vi "AlphaBetaToDQ_noSine.vi"(0 "alpha":sgl format="%#_32g", 1 "cosx":sgl, 2 "sinx":sgl, 5 "beta":sgl format="%#_32g", 12 "Resources":T1) -> (4 "direct":sgl, 6 "quadrature":sgl)   [LabVIEW 2017]
uses:
  Multiplier/Multiplier.lvclass
  Adder/Adder.lvclass
  Subtractor/Subtractor.lvclass
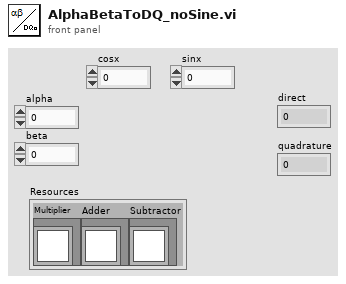
[diagram p1: front panel]
types:
  T1 = cluster{"Multiplier":refnum<class "Multiplier.lvclass">, "Adder":refnum<class "Adder.lvclass">, "Subtractor":refnum<class "Subtractor.lvclass">}
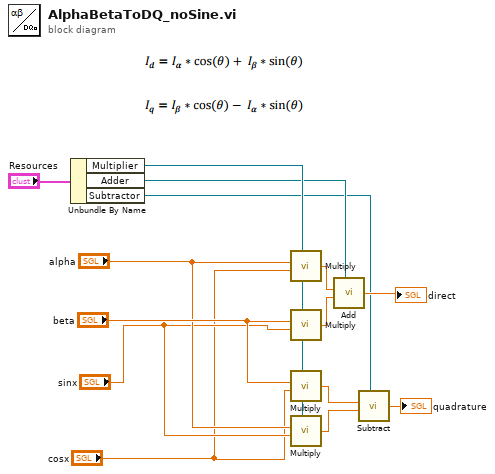
[diagram p0: block diagram]
diagram:
  n1 = Unbundle By Name("Resources") -> ("Multiplier"=w9:refnum<class "Multiplier.lvclass">, "Adder"=w2:refnum<class "Adder.lvclass">, "Subtractor"=w1:refnum<class "Subtractor.lvclass">)
  n2 = call-dynamic "Multiply.vi"("x"="alpha", "y"="cosx", "Multiplier"=w9) -> ("x*y"=w7:sgl)  [unwired: 4 in]
  n3 = call-dynamic "Multiply.vi"("x"="beta", "y"="sinx", "Multiplier"=w9) -> ("x*y"=w6:sgl)  [unwired: 4 in]
  n4 = call-dynamic "Multiply.vi"("x"="beta", "y"="cosx", "Multiplier"=w9) -> ("x*y"=w5:sgl)  [unwired: 4 in]
  n5 = call-dynamic "Multiply.vi"("x"="alpha", "y"="sinx", "Multiplier"=w9) -> ("x*y"=w4:sgl)  [unwired: 4 in]
  n6 = call-dynamic "Add.vi"("x"=w7, "y"=w6, "Adder"=w2) -> ("x+y"=→"direct":sgl)  [unwired: 4 in]
  n7 = call-dynamic "Subtract.vi"("x"=w5, "y"=w4, "Subtractor"=w1) -> ("x-y"=→"quadrature":sgl)  [unwired: 4 in]
